vi "Rs232_Read-v2_with_elapse.vi"() -> ()   [LabVIEW 2018]
uses:
  <vilib>/Instr/_visa.llb/VISA Configure Serial Port (Instr).vi
panel:
  in  "Time Target (s)":dbl=1.0
  out "Waveform Chart":dbl(graph)
  out "number":dbl
  in  "stop":bool
  out "error out":errorcluster
  in  "VISA resource name":refnum<visa-resource-name>
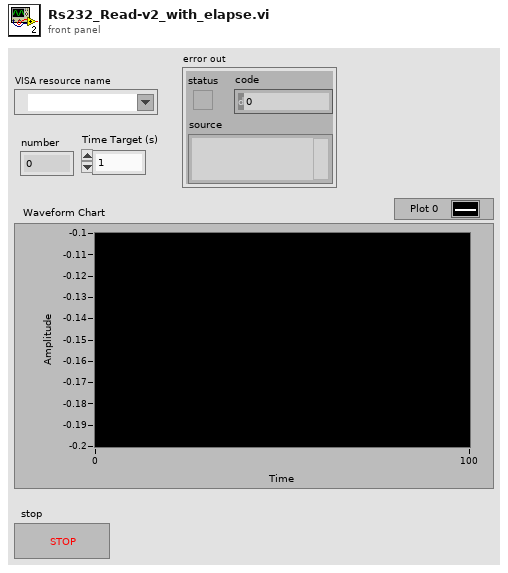
[diagram p1: front panel]
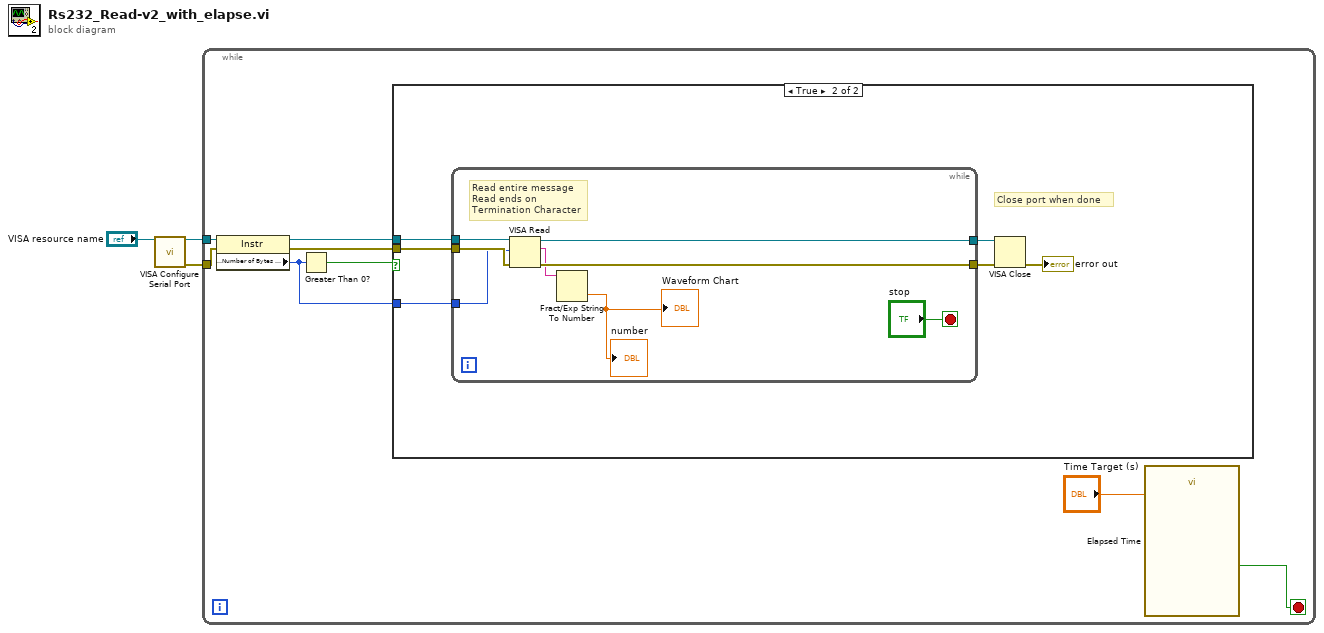
[diagram p0: block diagram]
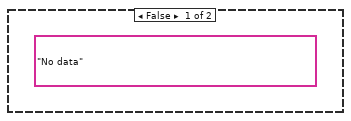
[diagram p2: hidden frame]
diagram:
  n1 = call-poly "VISA Configure Serial Port"("VISA resource name"="VISA resource name") -> ("VISA resource name out"=w2:refnum<visa-resource-name>, "error out"=w1:errorcluster)  [unwired: 13 in]
  n2 = while {
    tunnel: w2 -> [w11]
    tunnel: w1 -> [w10]
    stop <- w4 stop-if-true
    n3 = property class="Instr"(reference=w11, error in=w10) -> (reference out=w8:refnum<visa-resource-name>, error out=w7:errorcluster, "Serial Settings:Number of Bytes at Serial Port"=w6:u32)
    n4 = Greater Than 0?(x=w6) -> (x > 0?=w9:bool)
    n5 = case shown="True" w9 {
      tunnel: w8 -> [_ w14]
      tunnel: w7 -> [_ w13]
      tunnel: w6 -> [_ w12]
      frame False {
        (unwired) "No data"
      }
      frame True {
        # "Close port when done"
        n6 = while {
          tunnel: [w24] -> w16
          tunnel: [w23] -> w15
          tunnel: w14 -> [w20]
          tunnel: w13 -> [w19]
          tunnel: w12 -> [w18]
          stop <- "stop" stop-if-true
          # "Read entire message\nRead ends on\nTermination Character"
          n7 = VISA Read(VISA resource name=w20, byte count=w18, error in (no error)=w19) -> (VISA resource name out=w24:refnum<visa-resource-name>, read buffer=w22:string, error out=w23:errorcluster)  [unwired: 1 out]
          n8 = Fract/Exp String To Number(string=w22) -> (number=→"number" →"Waveform Chart":dbl)  [unwired: 3 in, 1 out]
        }
        n9 = VISA Close(VISA resource name=w16, error in (no error)=w15) -> (error out=→"error out":errorcluster)
      }
    }
    n10 = call "Elapsed Time"("Time Target (s)"="Time Target (s)") -> ("Time has Elapsed"=w4:bool)  [unwired: 11 in, 7 out]
  }
